vi "ClearBit.vi"(8 "error in (no error)":errorcluster, 10 "Index":i32, 11 "Prime_Sieve in":refnum<class "Prime_Sieve.lvclass">) -> (0 "error out":errorcluster, 3 "Prime_Sieve out":refnum<class "Prime_Sieve.lvclass">)   [LabVIEW 2020, in "Prime_Sieve.lvclass"]
uses:
  Prime_Sieve.lvclass
  Prime_Sieve.lvclass/Prime_Sieve.ctl
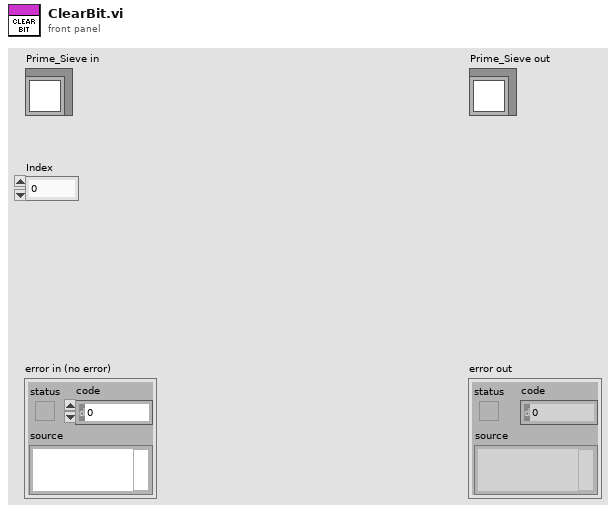
[diagram p1: front panel]
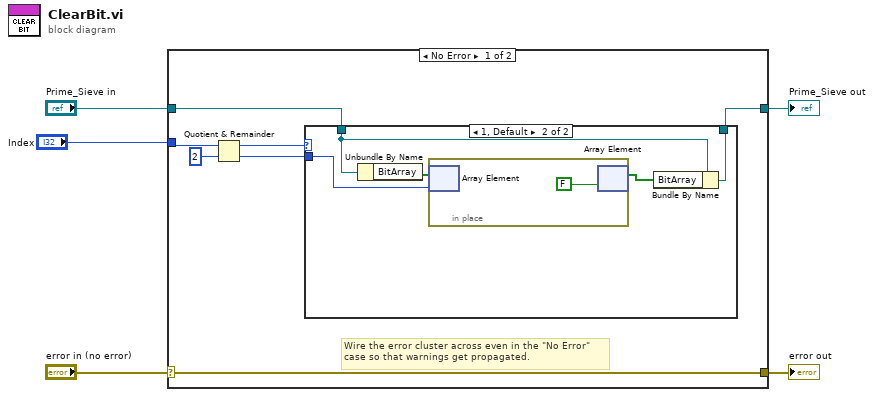
[diagram p0: block diagram]
diagram:
  n1 = case shown="No Error" "error in (no error)" {
    selector: "error in (no error)" -> [w12 w21]
    tunnel: [w12 w21] -> w4
    tunnel: [w9 w20] -> w2
    tunnel: "Prime_Sieve in" -> [w8 w20]
    tunnel: "Index" -> [w11 _]
    frame No Error {
      # "Wire the error cluster across even in the \"No Error\"\ncase so that warnings get propagated."
      n2 = Quotient & Remainder(x=w11, y=2) -> (x-y*floor(x/y)=w10:i32, floor(x/y)=w7:i32)
      n3 = case shown="1, Default" w10 {
        tunnel: w7 -> [_ w17]
        tunnel: w8 -> [w13 w16]
        tunnel: [w13 w14] -> w9
        frame 0 {
        }
        frame 1, Default {
          n4 = Unbundle By Name(w16) -> ("BitArray"=w18:bool[])
          n5 = in-place {
            n6 = in-place-array #1(w18, w17) -> ()  [unwired: 1 out]
            n7 = in-place-array #1(FALSE) -> (w15:bool[])  [unwired: 1 out]
          }
          n8 = Bundle By Name(cluster=w16, "BitArray"=w15) -> (w14:refnum<class "Prime_Sieve.lvclass">)
        }
      }
    }
    frame Error {
    }
  }
  "error out" <- w4
  "Prime_Sieve out" <- w2
